vi "Main.vi"   [LabVIEW 2020]
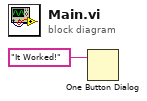
[diagram p0: block diagram]
diagram:
  n1 = One Button Dialog(message="It Worked!") -> ()  [unwired: 1 in, 1 out]
